vi "Curtin1_Colorize.vi"(9 "Instrument Notes":string, 11 "Text":refnum<vi>) -> ()   [LabVIEW 2022 SP3]
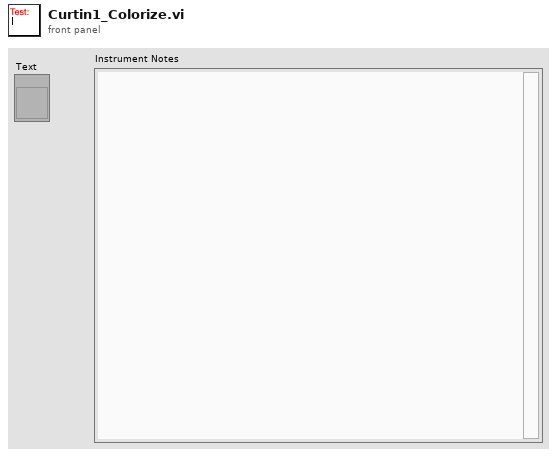
[diagram p1: front panel]
types:
  T1 = cluster{"offset past match":i32, "offset past match":i32}
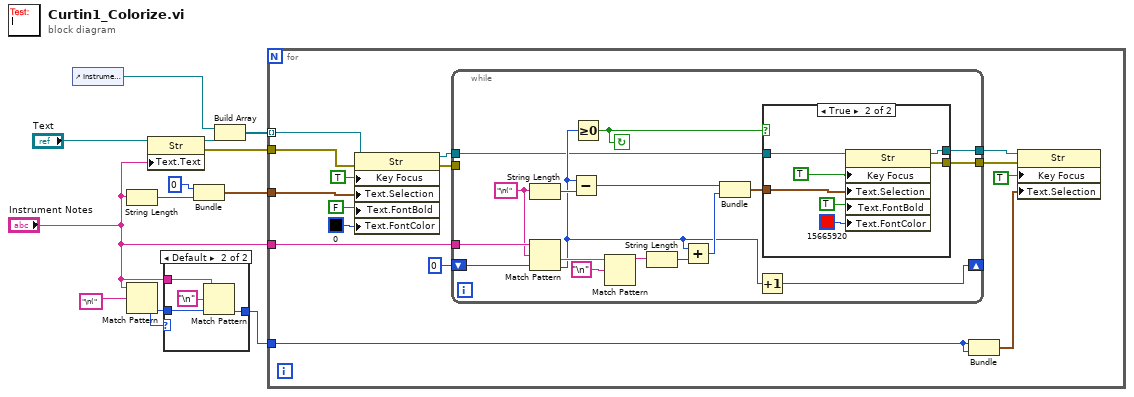
[diagram p0: block diagram]
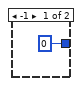
[diagram p2: hidden frame]
diagram:
  n1 = control-ref of="Instrument Notes"() -> (w6:refnum<vi>)
  n2 = String Length(string="Instrument Notes") -> (length=w12:i32)
  n3 = Match Pattern(string="Instrument Notes", regular expression="\n(") -> (offset past match=w3:i32)  [unwired: 1 in, 3 out]
  n4 = property class="Str"(reference="Text", "Text.Text"="Instrument Notes") -> (reference out=w7:refnum<vi>, error out=w8:errorcluster)  [unwired: 1 in]
  n5 = case shown="Default" w3 {
    tunnel: w3 -> [_ w17]
    tunnel: [0 ("offset past match") w15] -> w4
    tunnel: "Instrument Notes" -> [_ w14]
    frame -1 {
    }
    frame Default {
      n6 = Match Pattern(string=w14, regular expression="\n", offset (0)=w17) -> (offset past match=w15:i32)  [unwired: 3 out]
    }
  }
  n7 = Bundle(0, w12) -> (w11:cluster{i32, i32})  [unwired: 1 in]
  n8 = Build Array(w6, w7) -> (w5:refnum<vi>[])
  n9 = for {
    tunnel: w4 -> [w30]
    tunnel: w11 -> [w27]
    tunnel: "Instrument Notes" -> [w21]
    tunnel: w8 -> [w20]
    tunnel: w5 -> [w19] mode=indexing
    n10 = property on="Property Node" class="Str"(reference=w19, error in=w20, "Key Focus"=TRUE, "Text.Selection"=w27, "Text.FontBold"=FALSE ("Text.Font:Bold"), "Text.FontColor"=u32 0 ("Text.Text Colors:Text Color")) -> (reference out=w22:refnum<vi>, error out=w24:errorcluster)
    n11 = while {
      shift-right: [w47] -> _
      shift-left: 0 -> [w49]
      tunnel: w21 -> [w48]
      tunnel: [w35] -> w29
      tunnel: w24 -> [_]
      tunnel: [w34] -> w23
      tunnel: w22 -> [w33]
      stop <- w37 continue-if-true
      w43 = "\n(" ("regular expression")
      n12 = String Length(string=w43) -> (length=w44:i32)
      n13 = Match Pattern(string=w48, regular expression=w43, offset (0)=w49) -> (after substring=w46:string, offset past match=w36:i32)  [unwired: 2 out]
      n14 = Subtract(x=w36, y=w44) -> (x-y=w40:i32)
      n15 = Greater Or Equal To 0?(x=w36) -> (x >= 0?=w37:bool)
      n16 = Match Pattern(string=w46, regular expression="\n") -> (before substring=w42:string)  [unwired: 1 in, 3 out]
      n17 = String Length(string=w42) -> (length=w41:i32)
      n18 = Add(x=w36, y=w41) -> (x+y=w39:i32)
      n19 = Bundle(w40, w39) -> (w38:cluster{i32, i32})  [unwired: 1 in]
      n20 = Increment(x=w36) -> (x+1=w47:i32)
      n21 = case shown="True" w37 {
        tunnel: w38 -> [_ w56]
        tunnel: [_ w53] -> w35
        tunnel: [w50 w52] -> w34
        tunnel: w33 -> [w50 w51]
        frame False {
        }
        frame True {
          n22 = property on="Property Node" class="Str"(reference=w51, "Key Focus"=TRUE, "Text.Selection"=w56, "Text.FontBold"=TRUE ("Text.Font:Bold"), "Text.FontColor"=u32 15665920 ("Text.Text Colors:Text Color")) -> (reference out=w52:refnum<vi>, error out=w53:errorcluster)  [unwired: 1 in]
        }
      }
    }
    n23 = Bundle("offset past match"=w30, "offset past match"=w30) -> (w32:T1)  [unwired: 1 in]
    n24 = property on="Property Node" class="Str"(reference=w23, error in=w29, "Key Focus"=TRUE, "Text.Selection"=w32) -> ()  [unwired: 2 out]
  }
